vi "Signals to JSON 2.vi"() -> ()   [LabVIEW 2021]
uses:
  5eec69ea-4072-4200-a2f8-4861d0f2fd1f.vi
  <vilib>/JDP Science/JSONtext/Variant to JSON Text.vi
  <vilib>/JDP Science/JSONtext/LVClass Serializer/JSONtext LVClass Serializer.lvclass
panel:
  out "JSON string":string
  in  "Signal Sessions":T1
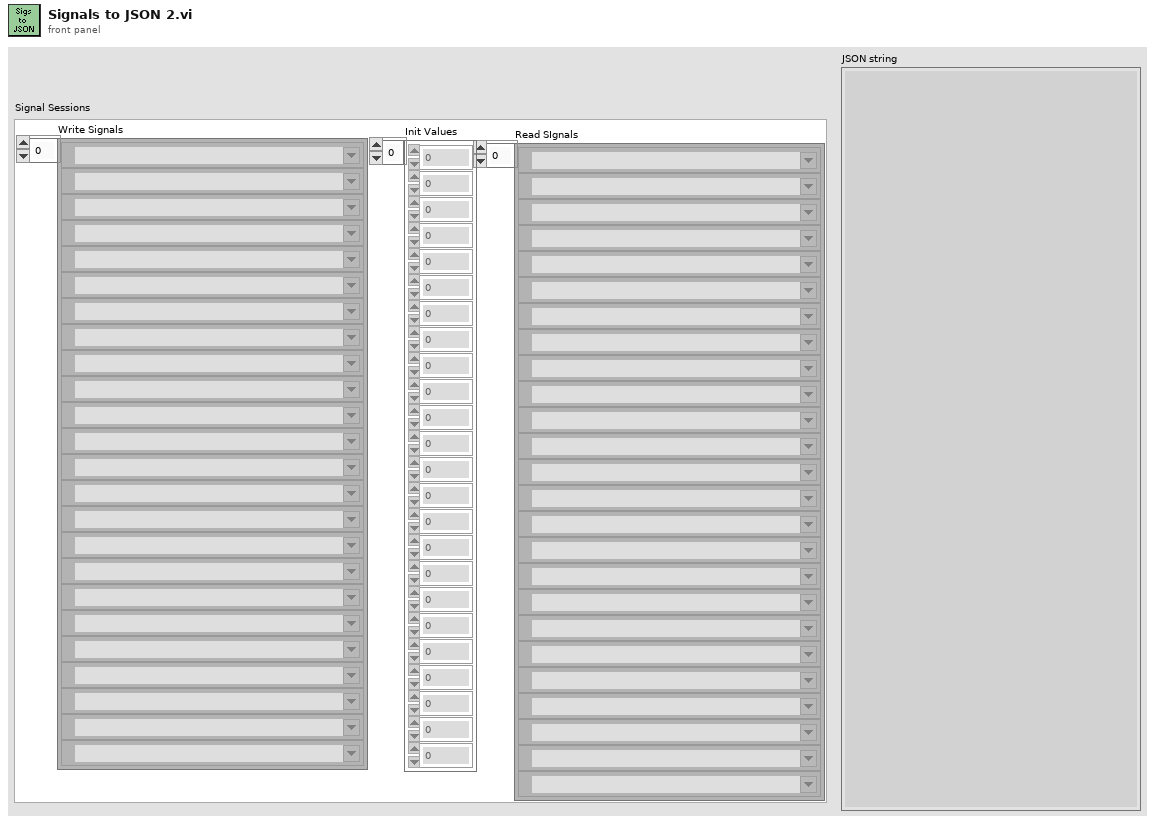
[diagram p1: front panel]
types:
  T1 = cluster{"Read SIgnals":refnum<k21>[], "Write Signals":refnum<k21>[], "Init Values":i32[]}
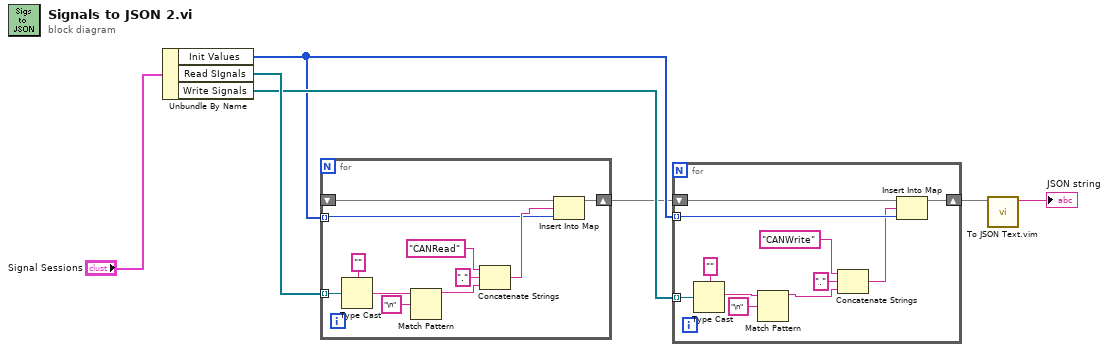
[diagram p0: block diagram]
diagram:
  n1 = Unbundle By Name("Signal Sessions") -> ("Init Values"=w4:i32[], "Read SIgnals"=w6:refnum<k21>[], "Write Signals"=w5:refnum<k21>[])
  n2 = for {
    tunnel: w6 -> [w17] mode=indexing
    tunnel: w4 -> [w10] mode=indexing
    shift-right: [w9] -> w2
    shift-left: _ -> [w8]
    n3 = Type Cast(type="", x=w17) -> (*(type *) &x=w14:string)
    n4 = Match Pattern(string=w14, regular expression="\n") -> (before substring=w12:string)  [unwired: 1 in, 3 out]
    n5 = Concatenate Strings("CANRead" ("type"), "." ("string"), w12) -> (w11:string)
    n6 = Insert Into Map(map in=w8, key=w11, value=w10) -> (map out=w9:map{string, i32})  [unwired: 2 out]
  }
  n7 = for {
    tunnel: w5 -> [w28] mode=indexing
    tunnel: w4 -> [w21] mode=indexing
    shift-right: [w19] -> w1
    shift-left: w2 -> [w22]
    n8 = Type Cast(type="", x=w28) -> (*(type *) &x=w24:string)
    n9 = Match Pattern(string=w24, regular expression="\n") -> (before substring=w23:string)  [unwired: 1 in, 3 out]
    n10 = Concatenate Strings("CANWrite" ("type"), "." ("string"), w23) -> (w20:string)
    n11 = Insert Into Map(map in=w22, key=w20, value=w21) -> (map out=w19:map{string, i32})  [unwired: 2 out]
  }
  n12 = call "To JSON Text.vim"("Anything"=w1) -> ("<JSON>"=→"JSON string":string)  [unwired: 9 in, 1 out]
